vi "PositionForceLoop.vi"() -> ()   [LabVIEW 2013]
panel:
  out "x/y":dbl
  in  "Actual Control Period (ticks)":u32
  in  "Sample Period (sec)":fxp<+/-,16,16>
  in  "Target Position x* (m)":fxp<+/-,16,16>
  in  "Target Force F*(N)":fxp<+/-,16,16>
  in  "Position FB x (m)":fxp<+/-,16,16>
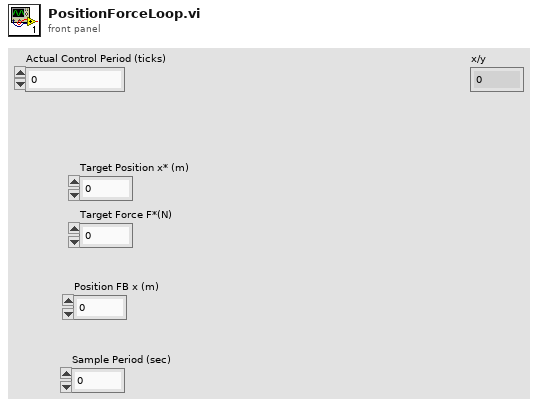
[diagram p1: front panel]
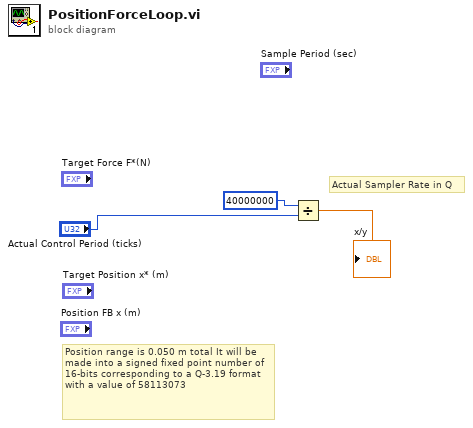
[diagram p0: block diagram]
diagram:
  # "Actual Sampler Rate in Q"
  # "Position range is 0.050 m total It will be made into a signed fixed point number of 16-bits corresponding to a Q-3.19 format with a value of 58113073"
  n1 = Divide(x=40000000, y="Actual Control Period (ticks)") -> (x/y=→"x/y":dbl)
